vi "stop.vi"(8 "error in (no error)":errorcluster) -> (0 "error out":errorcluster)   [LabVIEW 2015, in "lv-launcher-nre.lvlib"]
uses:
  lv-launcher-nre.lvlib
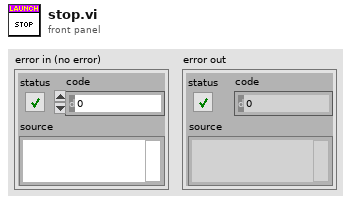
[diagram p1: front panel]
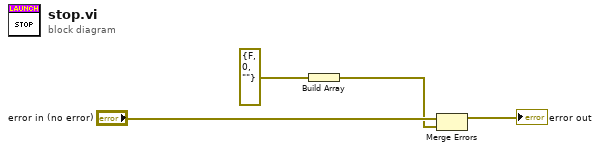
[diagram p0: block diagram]
diagram:
  n1 = Build Array(errorcluster {"status"=FALSE, "code"=0, "source"=""} ("error in (no error)")) -> (w2:errorcluster[])
  n2 = Merge Errors("error in (no error)", w2) -> (→"error out":errorcluster)
